vi "oa_Extract First Cycle Data (1 Channel).vi"(0 "resampled signal":cluster{"r0":dbl, "dr":dbl, "Y":dbl[]}={"r0"=0.0, "dr"=1.0, "Y"=[]} {"r0" format="%.2p"; "dr" format="%.2p"; "Y" format="%.2f"}, 1 "reset? (True)":bool=TRUE, 5 "speed profile":T1 {"speed [RPM]" format="%.2f"; "time [s]" format="%.2f"}, 7 "interpolated pulse positions":dbl[](array[numeric]) format="%.2f", 11 "error in (no error)":errorcluster) -> (4 "resampled signal out":cluster{"r0":dbl, "dr":dbl, "Y":dbl[]}={"r0"=0.0, "dr"=1.0, "Y"=[]} {"r0" format="%.2p"; "dr" format="%.2p"; "Y" format="%.2f"}, 6 "waveform reference data":cluster{"r0":dbl, "dr":dbl, "Y":dbl[]}={"r0"=0.0, "dr"=1.0, "Y"=[]} {"r0" format="%.2p"; "dr" format="%.2p"; "Y" format="%.2f"}, 15 "error out":errorcluster)   [LabVIEW 2017, in "SoundVib_RefDataProcess.lvlib"]
uses:
  <vilib>/addons/Sound and Vibration/Order Analysis/Referece Data Processing/SoundVib_RefDataProcess.lvlib
  <vilib>/addons/Sound and Vibration/Order Analysis/Tach Process/SubVIs/speed profile.ctl
  <vilib>/addons/Sound and Vibration/Order Analysis/Resample Order Tracking/SoundVib_Resampling.lvlib
  <vilib>/addons/Sound and Vibration/Order Analysis/Tach Process/SoundVib_TachProcess.lvlib
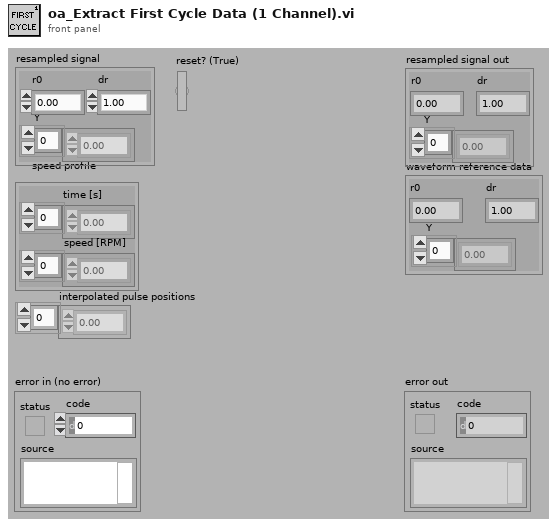
[diagram p1: front panel]
types:
  T1 = typedef "SoundVib_TachProcess.lvlib/speed profile.ctl" = cluster{"time [s]":dbl[], "speed [RPM]":dbl[]}
  T2 = enum16{"averaged samples", "initial samples", "final samples"}
  T3 = cluster{"r0":dbl, "dr":dbl, "reference data":dbl[]}
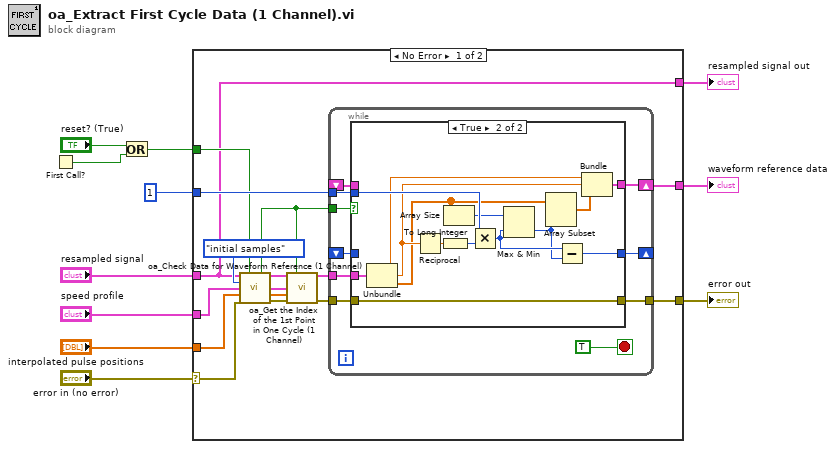
[diagram p0: block diagram]
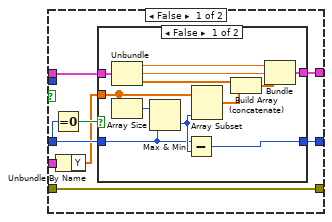
[diagram p2: hidden frame]
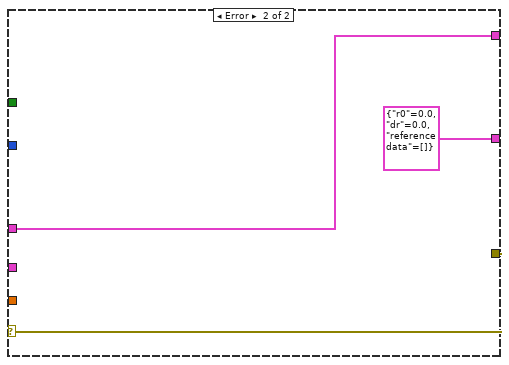
[diagram p4: hidden frame]
diagram:
  n1 = First Call?() -> (First Call?: T/F=w8:bool)
  n2 = Or(x="reset? (True)", y=w8) -> (x .or. y?=w7:bool)
  n3 = case shown="No Error" "error in (no error)" {
    selector: "error in (no error)" -> [w15 w76]
    tunnel: [w27 w76] -> w11
    tunnel: [w26 T3 {"r0"=0.0, "dr"=0.0, "reference data"=[]}] -> w10
    tunnel: 1 ("y") -> [w23 _]
    tunnel: w7 -> [w19 _]
    tunnel: "speed profile" -> [w18 _]
    tunnel: "resampled signal" -> [w12 w74]
    tunnel: "interpolated pulse positions" -> [w14 _]
    tunnel: [w12 w74] -> w1
    frame No Error {
      n4 = call <vilib>:"oa_Check Data for Waveform Reference (1 Channel).vi"("resampled signal"=w12, "reset? (True)"=w19, "select reference data"=T2."initial samples", "speed profile"=w18, "interpolated pulse positions"=w14, "error in (no error)"=w15) -> ("reset"=w20:bool, "resampled signal out"=w21:cluster{"r0":dbl, "dr":dbl, "Y":dbl[]}, "speed profile out"=w25:T1, "interpolated pulse positions out"=w24:dbl[], "error out"=w22:errorcluster)  [unwired: 2 in, 3 out]
      n5 = call <vilib>:"oa_Get the Index of the 1st Point in One Cycle (1 Channel).vi"("resampled signal"=w21, "reset? (True)"=w20, "speed profile"=w25, "interpolated pulse positions"=w24, "error in (no error)"=w22) -> ("resampled signal out"=w16:cluster{"r0":dbl, "dr":dbl, "Y":dbl[]}, "error out"=w17:errorcluster)  [unwired: 8 in, 1 out]
      n6 = while {
        tunnel: w20 -> [w37]
        tunnel: w17 -> [w36]
        tunnel: w23 -> [w34]
        shift-right: [w33] -> w26
        shift-left: _ -> [w31]
        shift-right: [w32] -> _
        shift-left: _ -> [w30]
        tunnel: [w29] -> w27
        tunnel: w16 -> [w28]
        stop <- TRUE stop-if-true
        n7 = case shown="True" w37 {
          tunnel: w36 -> [w40 w60]
          tunnel: w34 -> [_ w73]
          tunnel: [w41 w66] -> w33
          tunnel: [w45 w65] -> w32
          tunnel: w31 -> [w44 _]
          tunnel: w30 -> [w43 _]
          tunnel: [w40 w60] -> w29
          tunnel: w28 -> [w38 w61]
          frame False {
            n8 = Equal To 0?(x=w43) -> (x = 0?=w42:bool)
            n9 = Unbundle By Name(w38) -> ("Y"=w39:dbl[])
            n10 = case shown="False" w42 {
              tunnel: [w56 w58] -> w45
              tunnel: w39 -> [w55 _]
              tunnel: w44 -> [w53 w59]
              tunnel: w43 -> [w52 w58]
              tunnel: [w46 w59] -> w41
              frame False {
                n11 = Unbundle(w53) -> ("r0"=w47:dbl, "dr"=w48:dbl, w51:dbl[])
                n12 = Array Size(array=w55) -> (size(s)=w57:i32)
                n13 = Max & Min(x=w57, y=w52) -> (min(x,y)=w54:i32)  [unwired: 1 out]
                n14 = Subtract(x=w52, y=w54) -> (x-y=w56:i32)
                n15 = Array Subset(array=w55, length=w54) -> (w50:dbl[])  [unwired: 1 in]
                n16 = Build Array (concatenate)(w51, w50) -> (w49:dbl[])
                n17 = Bundle("r0"=w47, "dr"=w48, w49) -> (w46:cluster{"r0":dbl, "dr":dbl, dbl[]})  [unwired: 1 in]
              }
              frame True {
              }
            }
          }
          frame True {
            n18 = Unbundle(w61) -> ("r0"=w62:dbl, "dr"=w64:dbl, "Y"=w63:dbl[])
            n19 = Reciprocal(x=w64) -> (1/x=w72:dbl)
            n20 = To Long Integer(number=w72) -> (32bit integer=w71:i32)
            n21 = Array Size(array=w63) -> (size(s)=w70:i32)
            n22 = Multiply(x=w73, y=w71) -> (x*y=w69:i32)
            n23 = Max & Min(x=w70, y=w69) -> (min(x,y)=w68:i32)  [unwired: 1 out]
            n24 = Array Subset(array=w63, length=w68) -> (w67:dbl[])  [unwired: 1 in]
            n25 = Subtract(x=w69, y=w68) -> (x-y=w65:i32)
            n26 = Bundle("r0"=w62, "dr"=w64, w67) -> (w66:cluster{"r0":dbl, "dr":dbl, dbl[]})  [unwired: 1 in]
          }
        }
      }
    }
    frame Error {
    }
  }
  "waveform reference data" <- w10
  "error out" <- w11
  "resampled signal out" <- w1
